vi "close.vi"(8 "error in (no error)":errorcluster, 11 "ProEM_WinX32 in":refnum<class "ProEM_WinX32.lvclass">) -> (0 "error out":errorcluster)   [LabVIEW 2009, in "Hardware.lvlib" / "Channels.lvlib" / "ProEM_WinX32.lvclass"]
uses:
  ProEM_WinX32.lvclass
  ProEM_WinX32.lvclass/ProEM_WinX32.ctl
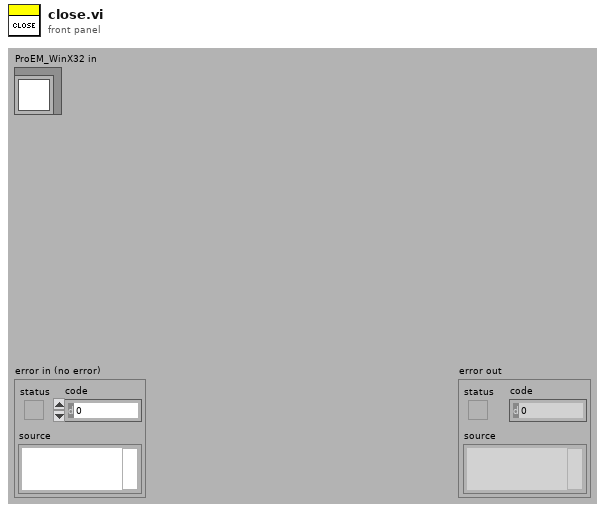
[diagram p1: front panel]
types:
  T1 = typedef "WINX32 Object Reference.ctl" = refnum<k1>
  T2 = typedef "WINX32 Data Members.ctl" = cluster{"WINX32Lib.IExpSetup":refnum<k7>, "WINX32Lib.IDocFile":refnum<k7>, "Result Image":T3, "Image to save":T3, "hardware present":bool, "started?":bool, "Image array from WINX":u16[][][], "raw images":cluster{"2D Image Array":u16[][]}[], "Camera active":bool, "images":T4, "Camera":T5}
  T3 = typedef "IMAQ Image.ctl" = refnum<image>
  T4 = typedef "WINX32 Image.ctl" = cluster{"processed":cluster{"Image":T3, u32}, "object":cluster{"Image":T3, u32}, "background":cluster{"Image":T3, u32}, "reference":cluster{"Image":T3, u32}, "mask":cluster{"Image":T3, u32}, "ROI Descriptor":cluster{"Global Rectangle":i32[], "Contours":cluster{"ID":enum32{"External", "Internal"}, "Type":enum32{"No Selection", "Point", "Line", "Rectangle", "Oval", "Polygon", "Free", "Unused1", "Unused2", "Unused3", "Broken Line", "Free Hand Line"}, "Coordinates":i32[]}[]}}
  T5 = typedef "Analyse - Camera.ctl" = cluster{"Bit Range(1023)":u32, "step(1.88)":dbl}
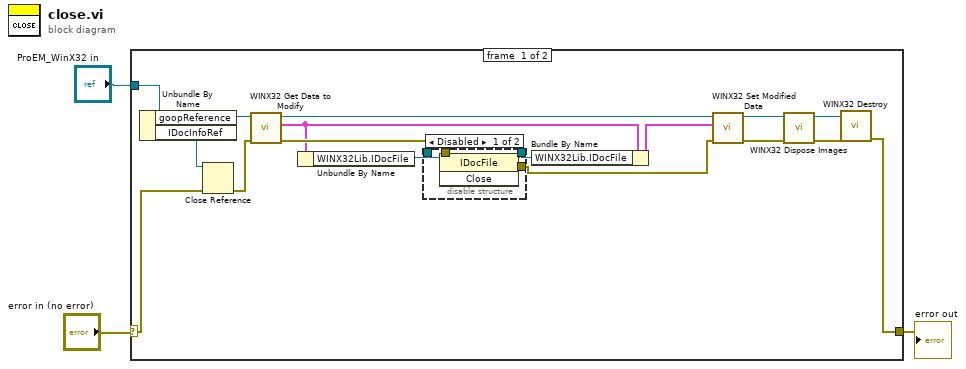
[diagram p0: block diagram]
diagram:
  n1 = case shown="No Error" "error in (no error)" {
    selector: "error in (no error)" -> [w4 w27]
    tunnel: "ProEM_WinX32 in" -> [w20 _]
    tunnel: [w16 w27] -> w1
    frame #0 {
      n2 = Unbundle By Name(w20) -> ("goopReference"=w19:T1, "IDocInfoRef"=w5:refnum<k7>)
      n3 = Close Reference(reference=w5, error in (no error)=w4) -> (error out=w6:errorcluster)
      n4 = call <instrlib>:"WINX32 Get Data to Modify.vi"("error in (no error)"=w6, "reference"=w19) -> ("error out"=w13:errorcluster, "data"=w12:T2, "duplicate reference"=w15:T1)  [unwired: 2 in, 1 out]
      n5 = Unbundle By Name(w12) -> ("WINX32Lib.IDocFile"=w14:refnum<k7>)
      n6 = disable-structure shown="Disabled" {
        disable-tunnel: w14 -> [w24 w26]
        disable-tunnel: w13 -> [w23 w25]
        disable-tunnel: [w22 w26] -> w11
        disable-tunnel: [w21 w25] -> w8
        frame #0 {
          n7 = invoke class="IDocFile" method="Close"(reference=w24, error in=w23) -> (reference out=w22:refnum<k7>, error out=w21:errorcluster)  [unwired: 1 in, 1 out]
        }
        frame #1 {
        }
      }
      n8 = Bundle By Name(cluster=w12, "WINX32Lib.IDocFile"=w11) -> (w9:T2)
      n9 = call <instrlib>:"WINX32 Set Modified Data.vi"("error in (no error)"=w8, "data"=w9, "reference"=w15) -> ("error out"=w7:errorcluster, "duplicate reference"=w10:T1)  [unwired: 3 in]
      n10 = call <instrlib>:"WINX32 Dispose Images.vi"("error in (no error)"=w7, "reference"=w10) -> ("error out"=w18:errorcluster, "duplicate reference"=w17:T1)  [unwired: 8 in]
      n11 = call <instrlib>:"WINX32 Destroy.vi"("error in (no error)"=w18, "reference"=w17) -> ("error out"=w16:errorcluster)  [unwired: 5 in]
    }
    frame #1 {
    }
  }
  "error out" <- w1
